vi "Write(Variant).vi"(6 "write to Cache only? (F)":bool, 7 "Qualified Name":string, 8 "error in (no error)":errorcluster, 9 "Name (empty: value name)":string, 10 "value":variant, 11 "ConfigManager in":refnum<class "ConfigManager.lvclass">) -> (0 "error out":errorcluster, 2 "keys written":string[](array[string]), 3 "ConfigManager out":refnum<class "ConfigManager.lvclass">)   [LabVIEW 2013, in "CfgManager.lvlib" / "ConfigManager.lvclass"]
uses:
  ConfigManager.lvclass
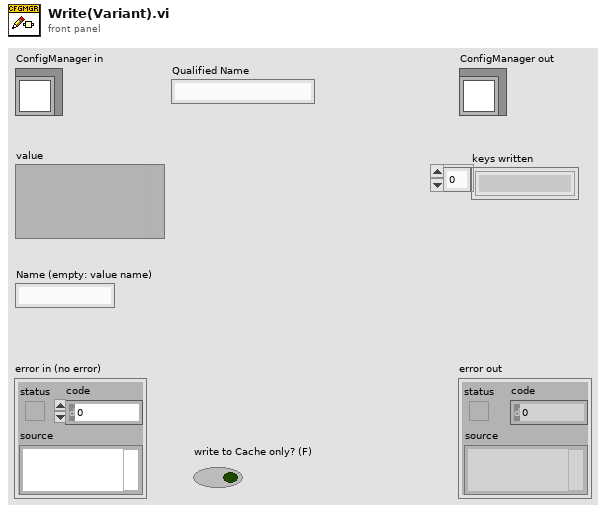
[diagram p1: front panel]
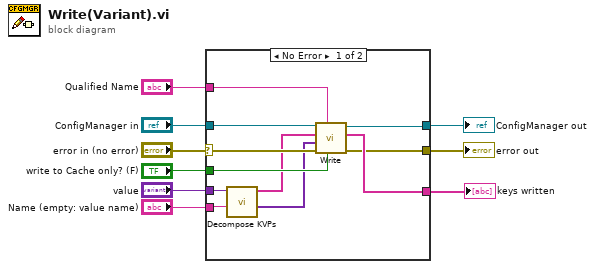
[diagram p0: block diagram]
diagram:
  n1 = case shown="No Error" "error in (no error)" {
    selector: "error in (no error)" -> [w16 w22]
    tunnel: [w15 w22] -> w6
    tunnel: [w18 w21] -> w8
    tunnel: "ConfigManager in" -> [w20 w21]
    tunnel: "Name (empty: value name)" -> [w11 _]
    tunnel: "value" -> [w13 _]
    tunnel: [w17 _] -> w3
    tunnel: "Qualified Name" -> [w19 _]
    tunnel: "write to Cache only? (F)" -> [w14 _]
    frame No Error {
      n2 = call "Decompose KVPs.vi"("Name (empty: value name)"=w11, "value"=w13) -> ("Values"=w12:variant[], "Keys"=w10:string[])  [unwired: 8 in]
      n3 = call "Write.vi"("write to Cache only? (F)"=w14, "Qualified Name"=w19, "error in (no error)"=w16, "Values"=w12, "keys"=w10, "ConfigManager in"=w20) -> ("error out"=w15:errorcluster, "keys dup"=w17:string[], "ConfigManager out"=w18:refnum<class "ConfigManager.lvclass">)  [unwired: 3 in]
    }
    frame Error {
    }
  }
  "error out" <- w6
  "ConfigManager out" <- w8
  "keys written" <- w3
